vi "Resize.Align Ctrl within Tab Ctrl.vi"(4 "Child Ref Pos":T1(ring), 5 "dY":i32, 6 "Parent Ref Pos":T1(ring), 7 "dX":i32, 8 "error in":errorcluster, 10 "Child Ctrl":refnum<vi>, 11 "Parent Tab Ctrl":refnum<vi>) -> (0 "error out":errorcluster, 2 "Child Ctrl Out":refnum<vi>, 3 "Parent Tab Ctrl Out":refnum<vi>)   [LabVIEW 2024, in "EQMF.lvlib" / "Controls.lvlib"]
uses:
  Controls.lvlib
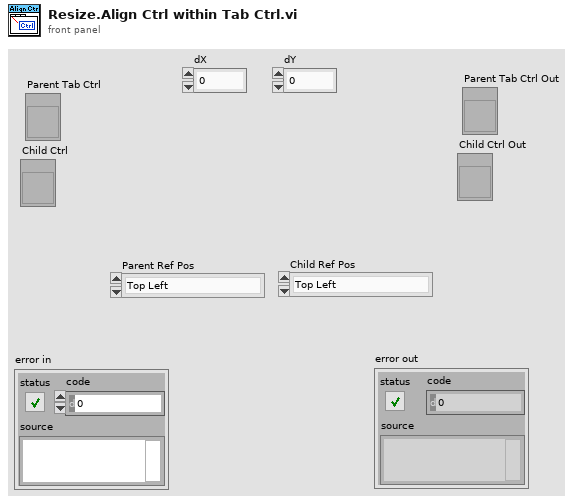
[diagram p1: front panel]
types:
  T1 = enum16{"Top Left", "Top Right", "Bottom Left", "Bottom Right"}
  T2 = typedef "EQMF.lvlib/Controls.lvlib/Ctrl.Object Position Info.ctl" = cluster{"Left":i32, "Right":i32, "Width":i32, "Top":i32, "Bottom":i32, "Height":i32}
  T3 = typedef "EQMF.lvlib/Controls.lvlib/Resize, Object Position Info.ctl" = cluster{"Left":i32, "Right":i32, "Width":i32, "Top":i32, "Bottom":i32, "Height":i32}
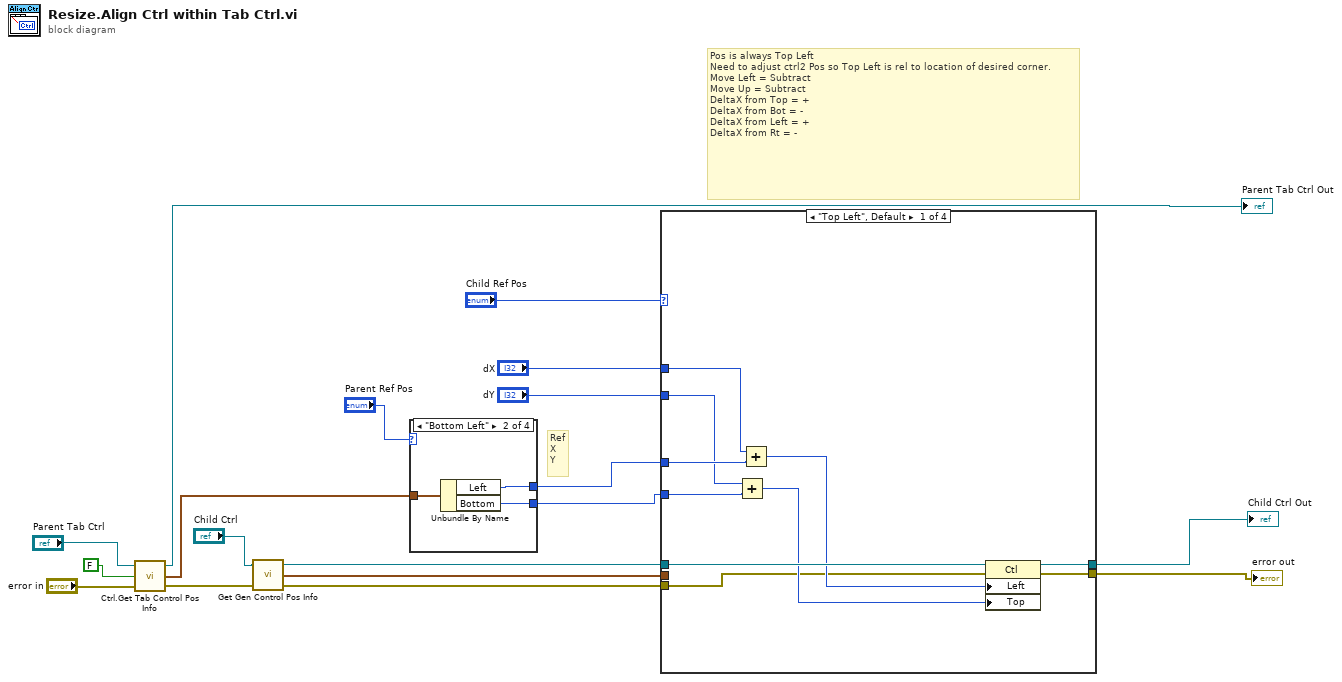
[diagram p0: block diagram]
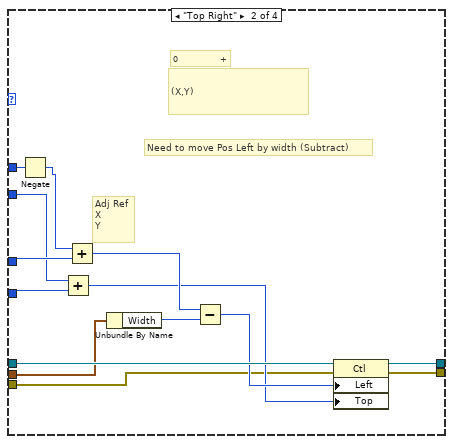
[diagram p2: hidden frame]
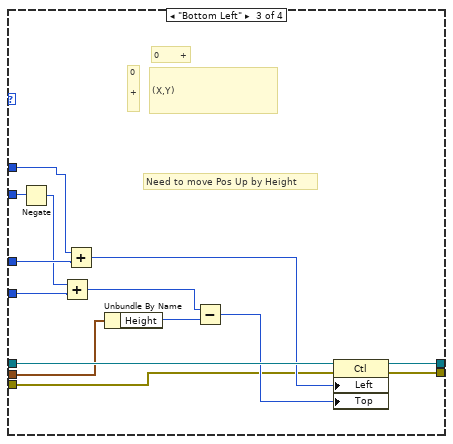
[diagram p3: hidden frame]
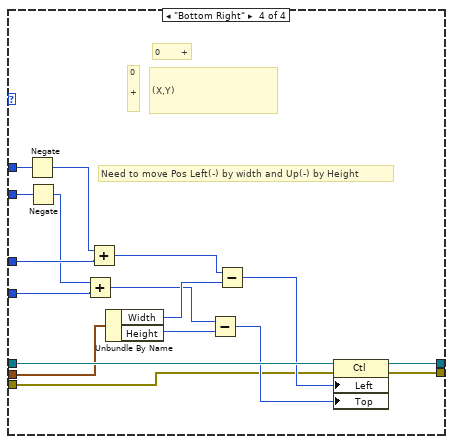
[diagram p4: hidden frame]
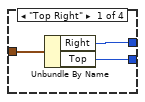
[diagram p5: hidden frame]
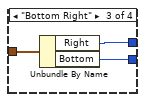
[diagram p6: hidden frame]
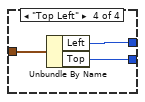
[diagram p7: hidden frame]
diagram:
  # "Pos is always Top Left\nNeed to adjust ctrl2 Pos so Top Left is rel to location of desired corner.\nMove Left = Subtract\nMove Up = Subtract\nDeltaX from Top = +\nDeltaX from Bot = -\nDeltaX from Left = +\nDeltaX from Rt = -"
  # "Ref\nX\nY"
  n1 = call "Ctrl.Get Tab Control Pos Info.vi"("error in"="error in", "Include Tab Height"=FALSE, "TabCtl Ref"="Parent Tab Ctrl") -> ("error out"=w4:errorcluster, "Pos Info"=w16:T2, "TabCtl Ref Out"=→"Parent Tab Ctrl Out":refnum<vi>)
  n2 = call "Get Gen Control Pos Info.vi"("error in"=w4, "Ctl Refnum"="Child Ctrl") -> ("error out"=w3:errorcluster, "Pos Info"=w14:T3, "Ctl Refnum Out"=w13:refnum<vi>)  [unwired: 1 in]
  n3 = case shown="\"Bottom Left\"" "Parent Ref Pos" {
    tunnel: w16 -> [w21 w24 w27 w30]
    tunnel: [w20 w23 w26 w29] -> w11
    tunnel: [w19 w22 w25 w28] -> w12
    frame "Top Right" {
      n4 = Unbundle By Name(w21) -> ("Right"=w20:i32, "Top"=w19:i32)
    }
    frame "Bottom Left" {
      n5 = Unbundle By Name(w24) -> ("Left"=w23:i32, "Bottom"=w22:i32)
    }
    frame "Bottom Right" {
      n6 = Unbundle By Name(w27) -> ("Right"=w26:i32, "Bottom"=w25:i32)
    }
    frame "Top Left" {
      n7 = Unbundle By Name(w30) -> ("Left"=w29:i32, "Top"=w28:i32)
    }
  }
  n8 = case shown="\"Top Left\", Default" "Child Ref Pos" {
    tunnel: w14 -> [_ w51 w65 w82]
    tunnel: w11 -> [w37 w47 w59 w76]
    tunnel: w12 -> [w36 w48 w61 w77]
    tunnel: w13 -> [w40 w54 w68 w85]
    tunnel: [w39 w53 w67 w84] -> w1
    tunnel: [w38 w52 w66 w83] -> w6
    tunnel: "dY" -> [w34 w46 w57 w71]
    tunnel: "dX" -> [w35 w43 w62 w73]
    tunnel: w3 -> [w31 w41 w55 w69]
    frame "Top Left", Default {
      n9 = Add(x=w34, y=w36) -> (x+y=w32:i32)
      n10 = Add(x=w35, y=w37) -> (x+y=w33:i32)
      n11 = property class="Ctl"(reference=w40, error in=w31, "Left"=w33, "Top"=w32) -> (reference out=w39:refnum<vi>, error out=w38:errorcluster)
    }
    frame "Top Right" {
      # "Adj Ref\nX\nY"
      # "0              +"
      # "Need to move Pos Left by width (Subtract)"
      # "(X,Y)"
      n12 = Negate(x=w43) -> (-x=w42:i32)
      n13 = Add(x=w46, y=w48) -> (x+y=w44:i32)
      n14 = Add(x=w42, y=w47) -> (x+y=w45:i32)
      n15 = Unbundle By Name(w51) -> ("Width"=w50:i32)
      n16 = Subtract(x=w45, y=w50) -> (x-y=w49:i32)
      n17 = property class="Ctl"(reference=w54, error in=w41, "Left"=w49, "Top"=w44) -> (reference out=w53:refnum<vi>, error out=w52:errorcluster)
    }
    frame "Bottom Left" {
      # "0       +"
      # "0\n\n+"
      # "Need to move Pos Up by Height"
      # "(X,Y)"
      n18 = Negate(x=w57) -> (-x=w56:i32)
      n19 = Add(x=w56, y=w61) -> (x+y=w60:i32)
      n20 = Add(x=w62, y=w59) -> (x+y=w58:i32)
      n21 = Unbundle By Name(w65) -> ("Height"=w64:i32)
      n22 = Subtract(x=w60, y=w64) -> (x-y=w63:i32)
      n23 = property class="Ctl"(reference=w68, error in=w55, "Left"=w58, "Top"=w63) -> (reference out=w67:refnum<vi>, error out=w66:errorcluster)
    }
    frame "Bottom Right" {
      # "0       +"
      # "0\n\n+"
      # "Need to move Pos Left(-) by width and Up(-) by Height"
      # "(X,Y)"
      n24 = Negate(x=w73) -> (-x=w72:i32)
      n25 = Negate(x=w71) -> (-x=w70:i32)
      n26 = Add(x=w70, y=w77) -> (x+y=w75:i32)
      n27 = Add(x=w72, y=w76) -> (x+y=w74:i32)
      n28 = Unbundle By Name(w82) -> ("Width"=w79:i32, "Height"=w81:i32)
      n29 = Subtract(x=w75, y=w81) -> (x-y=w80:i32)
      n30 = Subtract(x=w74, y=w79) -> (x-y=w78:i32)
      n31 = property class="Ctl"(reference=w85, error in=w69, "Left"=w78, "Top"=w80) -> (reference out=w84:refnum<vi>, error out=w83:errorcluster)
    }
  }
  "error out" <- w6
  "Child Ctrl Out" <- w1
